vi "Create DAQ RawDataQs.vi"(8 "error in (no error)":errorcluster, 10 "Accessors:AI TaskNames*":string[](array[string]), 11 "DAQ in":refnum<class "DAQ.lvclass">) -> (0 "error out":errorcluster, 2 "Variant":variant, 3 "DAQ out":refnum<class "DAQ.lvclass">)   [LabVIEW 2017, in "DAQ.lvclass"]
doc: "Developed by Kevin Thompson\nkevin@thompsonengineering.net\n\nCopyright 2018-2020\nThompson Engineering, LLC"
uses:
  DAQ.lvclass
  Process/ProcessSupport/TD local raw AI Data--cluster.ctl
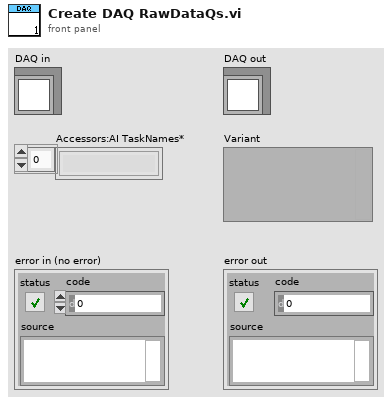
[diagram p1: front panel]
types:
  T1 = typedef "DAQ.lvclass/TD local raw AI Data--cluster.ctl" = cluster{"TimeStamp_(s)":dbl, "data":dbl[][]}
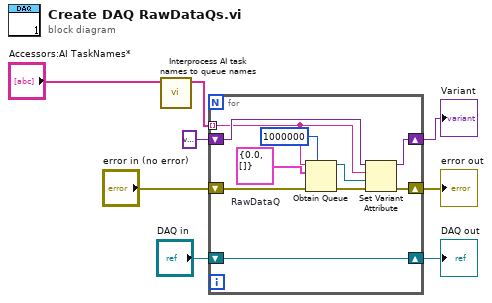
[diagram p0: block diagram]
diagram:
  n1 = call "Interprocess AI task names to queue names.vi"("Accessors:AI TaskNames*"="Accessors:AI TaskNames*") -> ("All Queues"=w1:string[])  [unwired: 8 in, 2 out]
  n2 = for {
    shift-right: [w11] -> w8
    shift-left: "error in (no error)" -> [w17]
    shift-right: [w13] -> w4
    shift-left: "DAQ in" -> [w13]
    tunnel: w1 -> [w10] mode=indexing
    shift-right: [w12] -> w5
    shift-left: variant ("Variant in") -> [w16]
    w18 = T1 {"TimeStamp_(s)"=0.0, "data"=[]}  # RawDataQ
    n3 = Obtain Queue(max queue size (-1, unlimited)=1000000, name (unnamed)=w10, element data type=w18, error in (no error)=w17) -> (queue out=w15:refnum<queue>, error out=w14:errorcluster)  [unwired: 1 in, 1 out]
    n4 = Set Variant Attribute(Variant=w16, name=w10, value=w15, error in=w14) -> (Variant out=w12:variant, error out=w11:errorcluster)  [unwired: 1 out]
  }
  "error out" <- w8
  "Variant" <- w5
  "DAQ out" <- w4
